vi "Create New Tree Item.vi"(7 "Item Type":T1=enum."Group", 8 "error in":errorcluster, 9 "found?":bool, 10 "index":i32, 11 "Left Cell String":string) -> (0 "error out":errorcluster, 3 "Item":T2)   [LabVIEW 2020, in "DSF Configuration Utility.lvlib"]
uses:
  DSF Configuration Utility.lvlib
  Tree Item.ctl
  ID to Tree Items/Tree Item Type.ctl
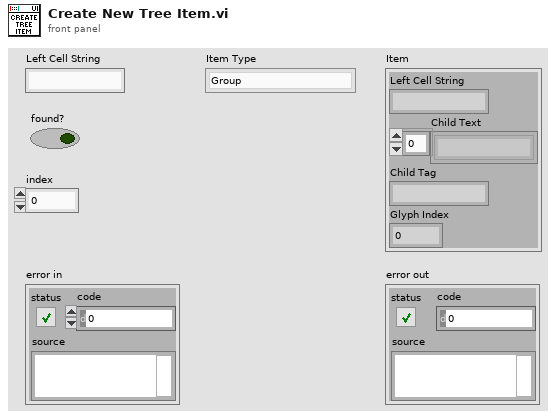
[diagram p1: front panel]
types:
  T1 = typedef "DSF Configuration Utility.lvlib/Tree Item Type.ctl" = enum16{"Plugin", "Group", "Transfer", "Channel", "Setting"}
  T2 = typedef "DSF Configuration Utility.lvlib/Tree Item.ctl" = cluster{"Left Cell String":string, "Child Text":string[], "Child Tag":string, "Glyph Index":i32}
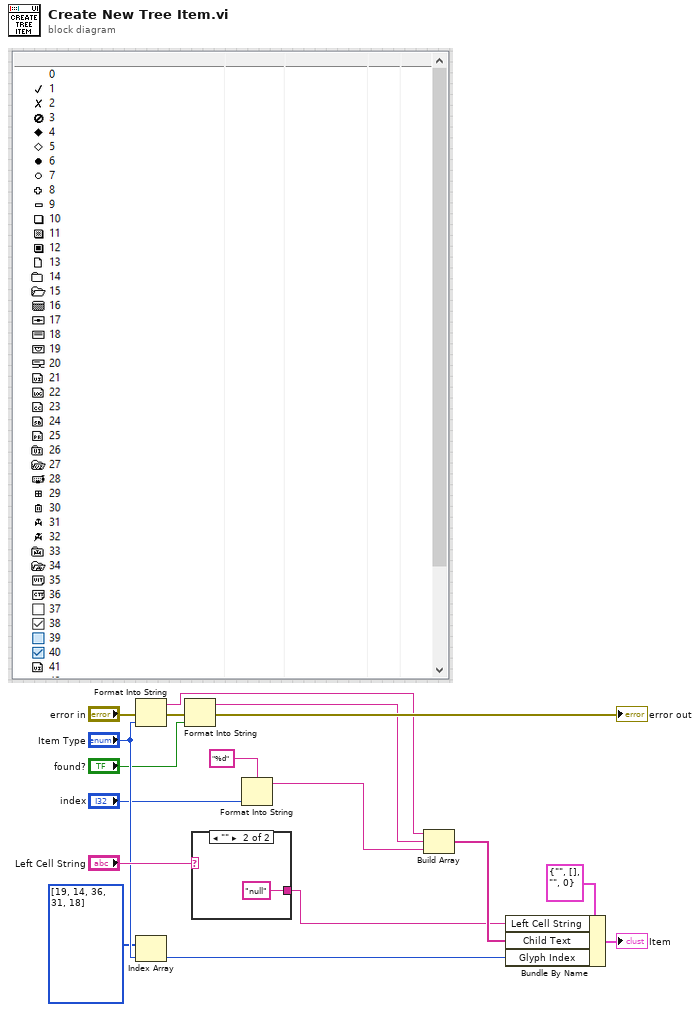
[diagram p0: block diagram]
diagram:
  n1 = Format Into String(error in="error in", "Item Type") -> (resulting string=w4:string, error out=w13:errorcluster)  [unwired: 2 in]
  n2 = Index Array(array=i32[] [19, 14, 36, 31, 18] ("f"), index="Item Type") -> (element=w7:i32)
  n3 = Format Into String(error in=w13, "found?") -> (resulting string=w5:string, error out=→"error out":errorcluster)  [unwired: 2 in]
  n4 = case shown="\"\"" "Left Cell String" {
    selector: "Left Cell String" -> [w18 _]
    tunnel: [w18 "null"] -> w10
    frame Default {
    }
    frame "" {
    }
  }
  n5 = Format Into String(format string="%d", "index") -> (resulting string=w1:string)  [unwired: 2 in, 1 out]
  n6 = Build Array(w4, w5, w1) -> (w16:string[])
  n7 = Bundle By Name(cluster=T2 {"Left Cell String"="", "Child Text"=[], "Child Tag"="", "Glyph Index"=0} ("Item"), "Left Cell String"=w10, "Child Text"=w16, "Glyph Index"=w7) -> (→"Item":T2)
